vi "read-current.vi"(3 "error in":errorcluster, 4 "Reset":bool, 5 "VISA resource name":refnum<visa-resource-name>="GPIB0::29::INSTR") -> (0 "error out":errorcluster, 1 "Raw output":string, 2 "Current (A)":dbl)   [LabVIEW 2013]
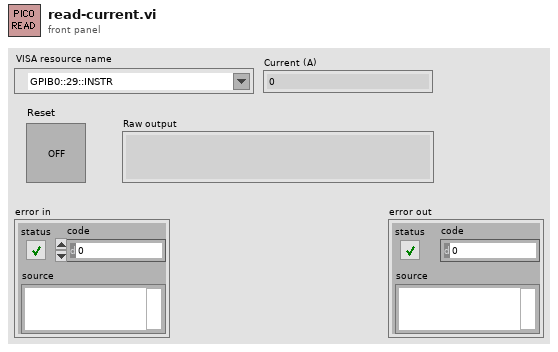
[diagram p1: front panel]
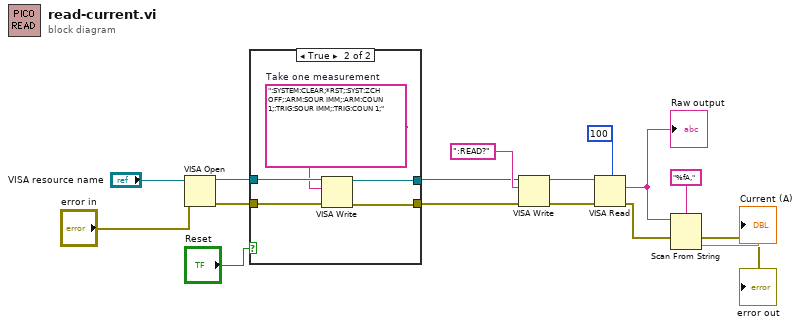
[diagram p0: block diagram]
diagram:
  n1 = VISA Open(error in (no error)="error in", VISA resource name="VISA resource name") -> (VISA resource name=w11:refnum<visa-resource-name>, error out=w8:errorcluster)  [unwired: 3 in]
  n2 = case shown="True" "Reset" {
    tunnel: w11 -> [w17 w23]
    tunnel: [w17 w21] -> w10
    tunnel: [w18 w19] -> w9
    tunnel: w8 -> [w18 w20]
    frame False {
    }
    frame True {
      w22 = ":SYSTEM:CLEAR;*RST;:SYST:ZCH OFF;:ARM:SOUR IMM;:ARM:COUN 1;:TRIG:SOUR IMM;:TRIG:COUN 1;"  # Take one measurement
      n3 = VISA Write(VISA resource name=w23, write buffer=w22, error in (no error)=w20) -> (VISA resource name out=w21:refnum<visa-resource-name>, error out=w19:errorcluster)  [unwired: 1 out]
    }
  }
  n4 = VISA Write(VISA resource name=w10, write buffer=":READ?", error in (no error)=w9) -> (VISA resource name out=w12:refnum<visa-resource-name>, error out=w7:errorcluster)  [unwired: 1 out]
  n5 = VISA Read(VISA resource name=w12, byte count=u32 100, error in (no error)=w7) -> (read buffer=w6:string, error out=w2:errorcluster)  [unwired: 2 out]
  "Raw output" <- w6
  n6 = Scan From String(format string="%fA," ("write buffer"), input string=w6, error in=w2) -> (error out=→"error out":errorcluster, output 1=→"Current (A)":dbl)  [unwired: 2 in, 2 out]
